vi "Run Stimulus Profile.vi"(6 "Timeout (s)":i32, 8 "uutSerialNumber":string, 9 "gatewayIP":string, 10 "file":string, 11 "Sequence Context In":refnum<k7>) -> (0 "error out":errorcluster, 2 "file out":string)   [LabVIEW 2015, in "RTSequenceVIs.lvlib"]
uses:
  RTSequenceVIs.lvlib
  NationalInstruments.VeriStand.RealTimeSequenceDefinitionApi
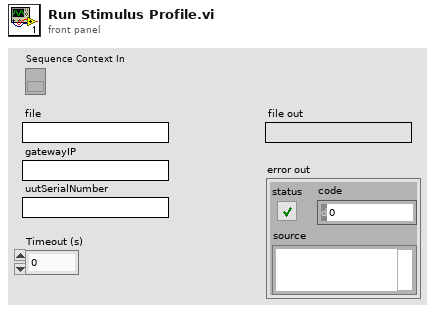
[diagram p1: front panel]
types:
  T1 = typedef "TestStand - Status Monitor.ctl" = cluster{"Sequence Context":refnum<k7>, "Execution":refnum<k7>, "Termination Monitor":refnum<k7>}
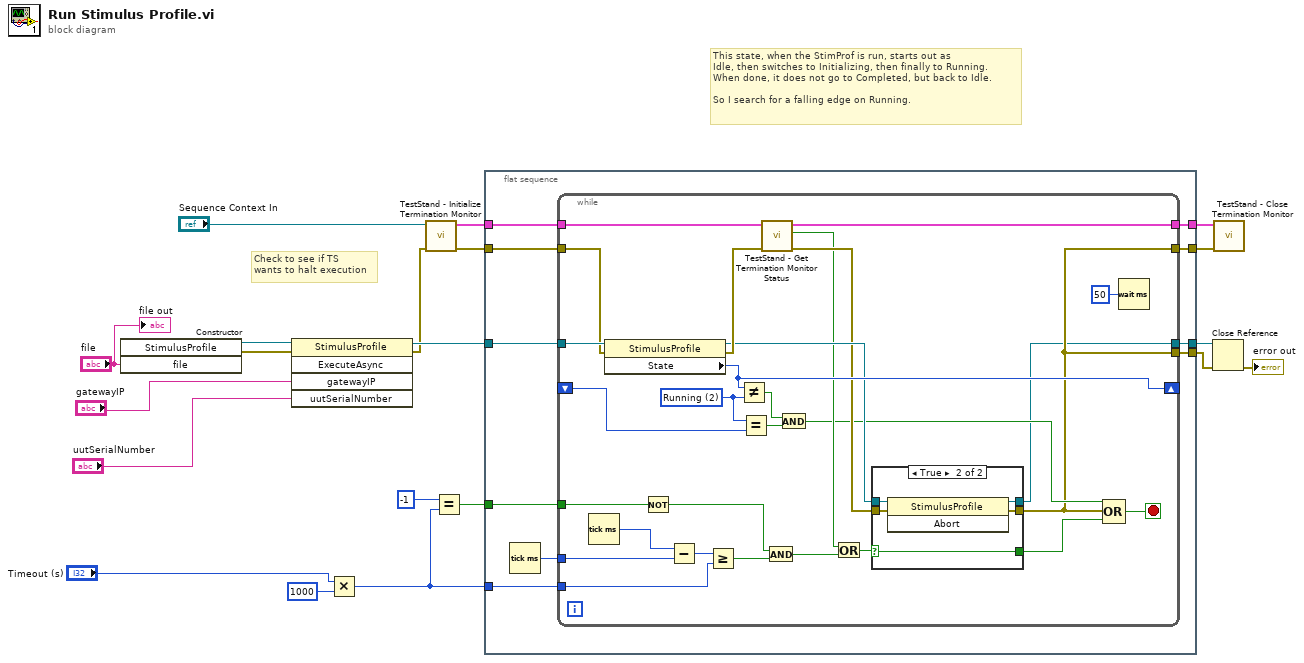
[diagram p0: block diagram]
diagram:
  # "Check to see if TS \nwants to halt execution"
  # "This state, when the StimProf is run, starts out as \nIdle, then switches to Initializing, then finally to Running.\nWhen done, it does not go to Completed, but back to Idle.\n\nSo I search for a falling edge on Running."
  n1 = constructor class="StimulusProfile"("file"="file") -> (reference out=w20:refnum<k24>, error out=w19:errorcluster)  [unwired: 3 in, 2 out]
  n2 = invoke class="StimulusProfile" method="ExecuteAsync"(reference=w20, error in=w19, "gatewayIP"="gatewayIP", "uutSerialNumber"="uutSerialNumber") -> (reference out=w16:refnum<k24>, error out=w7:errorcluster)  [unwired: 1 in, 3 out]
  n3 = Multiply(x="Timeout (s)", y=1000) -> (x*y=w3:i32)
  n4 = call <vilib>:"TestStand - Initialize Termination Monitor.vi"("error in (no error)"=w7, "Sequence Context In"="Sequence Context In") -> ("error out"=w8:errorcluster, "Status Monitor Out"=w11:T1)  [unwired: 8 in]
  n5 = Equal?(x=-1, y=w3) -> (x = y?=w2:bool)
  n6 = flat-sequence {
    tunnel: w16 -> [w30]
    tunnel: [w29] -> w15
    tunnel: [w28] -> w14
    tunnel: w11 -> [w27]
    tunnel: [w26] -> w10
    tunnel: [w25] -> w9
    tunnel: w8 -> [w24]
    tunnel: w3 -> [w23]
    tunnel: w2 -> [w22]
    frame #0 {
      n7 = Tick Count (ms)() -> (millisecond timer value=w21:u32)
      n8 = while {
        tunnel: w30 -> [w58]
        tunnel: [w31] -> w29
        tunnel: [w33] -> w28
        shift-right: [w56] -> _
        shift-left: _ -> [w54]
        tunnel: w27 -> [w50]
        tunnel: [w49] -> w26
        tunnel: [w33] -> w25
        tunnel: w24 -> [w47]
        tunnel: w23 -> [w42]
        tunnel: w22 -> [w46]
        tunnel: w21 -> [w44]
        stop <- w51 stop-if-true
        w55 = 2 items=["Idle", "Initializing", "Running", "Paused", "Finalizing", "Complete"] ("State")
        n9 = Tick Count (ms)() -> (millisecond timer value=w45:u32)
        n10 = property class="StimulusProfile"(reference=w58, error in=w47) -> (reference out=w39:refnum<k24>, error out=w48:errorcluster, "State"=w56:i32)
        n11 = Not(x=w46) -> (.not. x?=w41:bool)
        n12 = Subtract(x=w45, y=w44) -> (x-y=w43:u32)
        n13 = Greater Or Equal?(x=w43, y=w42) -> (x >= y?=w40:bool)
        n14 = Not Equal?(x=w56, y=w55) -> (x != y?=w53:bool)
        n15 = Equal?(x=w55, y=w54) -> (x = y?=w52:bool)
        n16 = call <vilib>:"TestStand - Get Termination Monitor Status.vi"("error in (no error)"=w48, "Status Monitor In"=w50) -> ("error out"=w38:errorcluster, "Terminating or Aborting"=w36:bool, "Status Monitor Out"=w49:T1)  [unwired: 7 in]
        n17 = And(x=w41, y=w40) -> (x .and. y?=w35:bool)
        n18 = And(x=w53, y=w52) -> (x .and. y?=w34:bool)
        n19 = Or(x=w36, y=w35) -> (x .or. y?=w37:bool)
        n20 = case shown="True" w37 {
          selector: w37 -> [_ w62]
          tunnel: w39 -> [w59 w65]
          tunnel: w38 -> [w60 w64]
          tunnel: [w60 w63] -> w33
          tunnel: [_ w62] -> w32
          tunnel: [w59 w61] -> w31
          frame False {
          }
          frame True {
            n21 = invoke class="StimulusProfile" method="Abort"(reference=w65, error in=w64) -> (reference out=w61:refnum<k24>, error out=w63:errorcluster)  [unwired: 1 in, 1 out]
          }
        }
        n22 = Compound Arithmetic op=OR(w34, w33, w32) -> (w51:bool)
        n23 = Wait (ms)(milliseconds to wait=u32 50) -> ()  [unwired: 1 out]
      }
    }
  }
  n24 = Close Reference(reference=w15, error in (no error)=w14) -> (error out=→"error out":errorcluster)
  n25 = call <vilib>:"TestStand - Close Termination Monitor.vi"("error in (no error)"=w9, "Status Monitor In"=w10) -> ()  [unwired: 9 in, 1 out]
  "file out" <- "file"
